vi "Sorry String Array.vi"(7 "Array of String":string[](array[string])) -> (8 "Sorted Array":string[](array[string]))   [LabVIEW 2016]
uses:
  <vilib>/regexp/Match Regular Expression.xnode
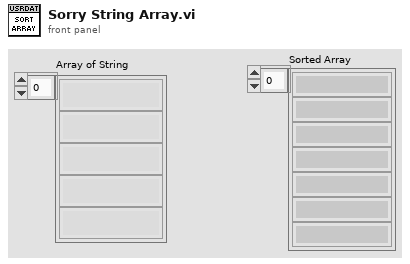
[diagram p1: front panel]
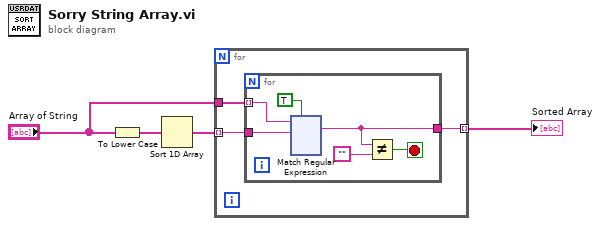
[diagram p0: block diagram]
diagram:
  n1 = To Lower Case(string="Array of String") -> (all lower case string=w4:string[])
  n2 = Sort 1D Array(array=w4) -> (sorted array=w3:string[])
  n3 = for {
    tunnel: w3 -> [w7] mode=indexing
    tunnel: "Array of String" -> [w5]
    tunnel: [w6] -> w1 mode=indexing
    n4 = for {
      tunnel: w7 -> [w13]
      tunnel: [w9] -> w6
      tunnel: w5 -> [w11] mode=indexing
      stop <- w10 stop-if-true
      n5 = xnode "Match Regular Expression"("input string"=w11, "regular expression"=w13, "ignore case? (F)"=TRUE) -> ("whole match"=w9:string)  [unwired: 3 in, 4 out]
      n6 = Not Equal?(x=w9, y="") -> (x != y?=w10:bool)
    }
  }
  "Sorted Array" <- w1
